vi "Calculate Distances.vi"(8 "error in (no error)":errorcluster, 11 "Grassfire in":refnum<class "Grassfire.lvclass">) -> (0 "error out":errorcluster, 3 "Grassfire out":refnum<class "Grassfire.lvclass">)   [LabVIEW 2019, in "Grassfire.lvclass"]
uses:
  Grassfire.lvclass
  Address/Address.lvclass
  Grassfire.lvclass/Grassfire.ctl
  Node/Node Value.lvclass
panel:
  out "i":i32
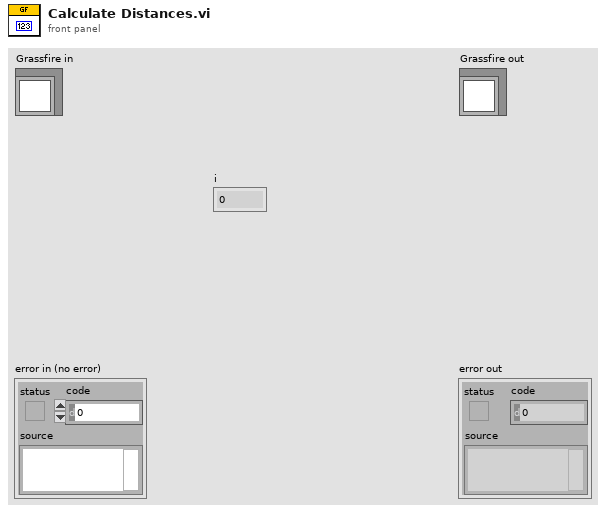
[diagram p1: front panel]
types:
  T1 = map{refnum<class "Address.lvclass">, refnum<class "Node Value.lvclass">}
  T2 = cluster{"Address":refnum<class "Address.lvclass">, "Step":i32}
  T3 = typedef "Node Value.lvclass/Node Type--enum.ctl" = enum16{"Empty", "Blocked", "Start", "End", "Path"}
  T4 = cluster{"2D Array Index":refnum<class "Address.lvclass">, i32}
  T5 = cluster{"Address":refnum<class "Address.lvclass">, "Step":i32}[]
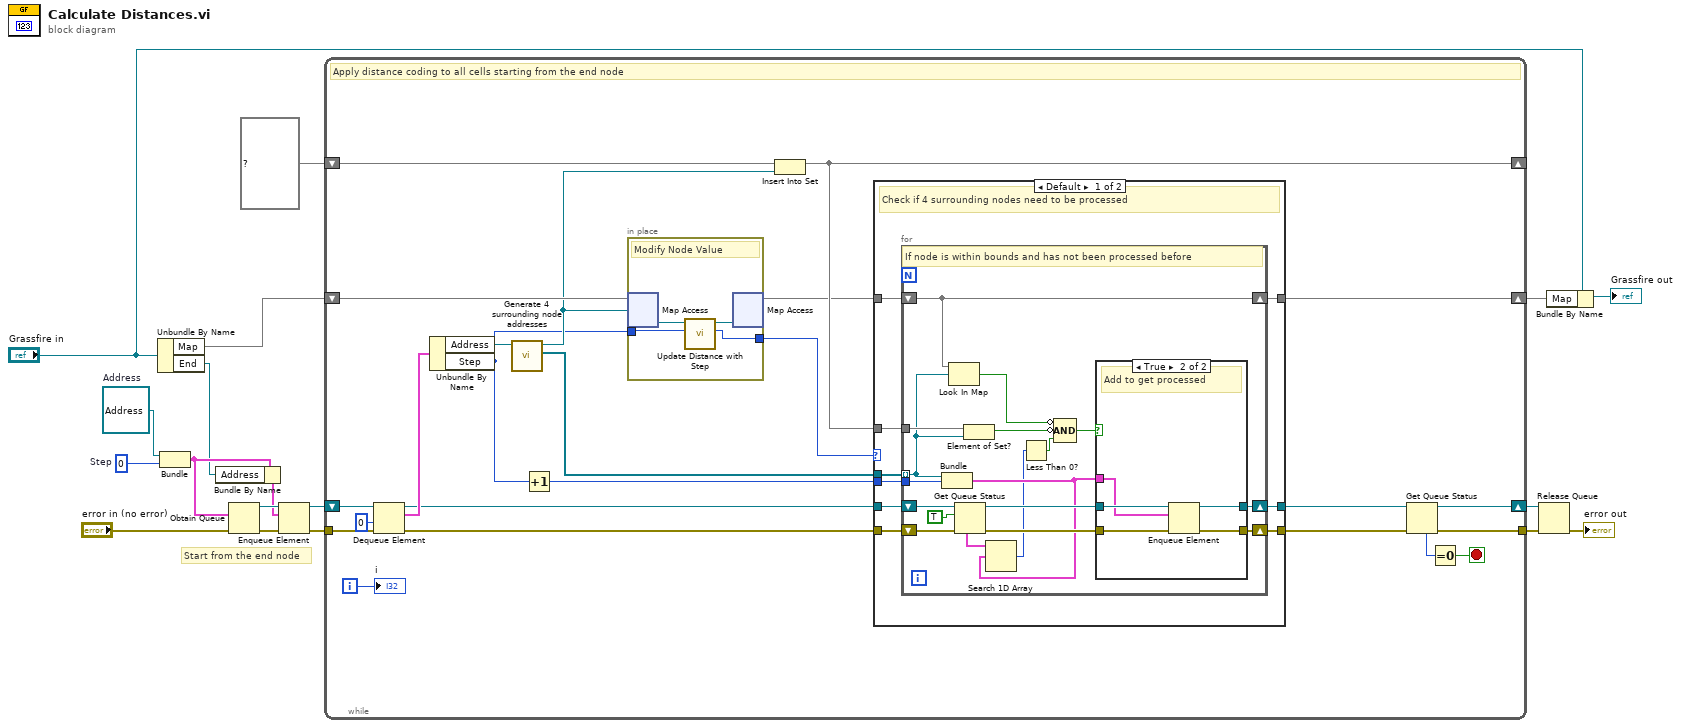
[diagram p0: block diagram]
diagram:
  w2 = refnum<class "Address.lvclass"> refnum  # Address
  w17 = 0  # Step
  # "Start from the end node"
  n1 = Unbundle By Name("Grassfire in") -> ("Map"=w12:T1, "End"=w14:refnum<class "Address.lvclass">)
  n2 = Bundle("Address"=w2, "Step"=w17) -> (w16:T2)  [unwired: 1 in]
  n3 = Bundle By Name(cluster=w16, "Address"=w14) -> (w15:T2)
  n4 = Obtain Queue(element data type=w16, error in (no error)="error in (no error)") -> (queue out=w18:refnum<queue>, error out=w9:errorcluster)  [unwired: 3 in, 1 out]
  n5 = Enqueue Element(queue=w18, element=w15, error in (no error)=w9) -> (queue out=w10:refnum<queue>, error out=w11:errorcluster)  [unwired: 1 in, 1 out]
  n6 = while {
    shift-right: [w42] -> w6
    shift-left: w12 -> [w25]
    shift-right: [w33] -> w4
    shift-left: w10 -> [w39]
    tunnel: w11 -> [w36]
    tunnel: [w34] -> w5
    shift-right: [w31] -> _
    shift-left: set{refnum<class "Address.lvclass">} {} ("set") -> [w32]
    i -> [w41]
    stop <- w30 stop-if-true
    # "Apply distance coding to all cells starting from the end node"
    n7 = Dequeue Element(queue=w39, timeout in ms (-1)=0, error in (no error)=w36) -> (queue out=w37:refnum<queue>, element=w38:T2, error out=w35:errorcluster)  [unwired: 1 out]
    n8 = Unbundle By Name(w38) -> ("Address"=w26:refnum<class "Address.lvclass">, "Step"=w20:i32)
    n9 = call "Generate 4 surrounding node addresses.vi"("2D Array in"=w26) -> ("4 Surrounding Nodes"=w23:refnum<class "Address.lvclass">[], "2D Array out"=w24:refnum<class "Address.lvclass">)  [unwired: 7 in, 2 out]
    n10 = Increment(x=w20) -> (x+1=w19:i32)
    n11 = in-place {
      in-place-border: w20 -> [w44]
      in-place-border: [w43] -> w22
      # "Modify Node Value"
      n12 = in-place-map #1(w25, w24) -> (w46:refnum<class "Node Value.lvclass">)  [unwired: 1 in, 1 out]
      n13 = call "Update Distance with Step.vi"("Step"=w44, "Picture Ring in"=w46) -> ("Node Type"=w43:T3, "Picture Ring out"=w45:refnum<class "Node Value.lvclass">)  [unwired: 7 in, 1 out]
      n14 = in-place-map #1(w45) -> (w21:T1)  [unwired: 1 in, 2 out]
    }
    n15 = Insert Into Set(10:w24, 11:w32) -> (3:w31:set{refnum<class "Address.lvclass">})  [unwired: 1 out]
    n16 = case shown="Default" w22 {
      tunnel: [w54 w82] -> w28
      tunnel: w23 -> [w53 _]
      tunnel: w37 -> [w55 w82]
      tunnel: w35 -> [w52 w81]
      tunnel: [w51 w81] -> w27
      tunnel: [w50 w83] -> w42
      tunnel: w21 -> [w49 w83]
      tunnel: w31 -> [w48 _]
      tunnel: w19 -> [w47 _]
      frame Default {
        # "Check if 4 surrounding nodes need to be processed"
        n17 = for {
          tunnel: w53 -> [w68] mode=indexing
          shift-right: [w73] -> w54
          shift-left: w55 -> [w65]
          shift-right: [w72] -> w51
          shift-left: w52 -> [w63]
          shift-right: [w66] -> w50
          shift-left: w49 -> [w66]
          tunnel: w48 -> [w69]
          tunnel: w47 -> [w59]
          # "If node is within bounds and has not been processed before"
          n18 = Bundle("2D Array Index"=w68, w59) -> (w58:T4)  [unwired: 1 in]
          n19 = Look In Map(map=w66, key=w68) -> (key not found?=w71:bool)  [unwired: 1 in, 1 out]
          n20 = Get Queue Status(queue=w65, return elements? (F)=TRUE, error in (no error)=w63) -> (queue out=w62:refnum<queue>, error out=w61:errorcluster, elements=w60:T5)  [unwired: 5 out]
          n21 = Element of Set?(10:w68, 11:w69) -> (3:w67:bool)
          n22 = Search 1D Array(1D array=w60, element=w58) -> (index of element=w56:i32)  [unwired: 1 in]
          n23 = Less Than 0?(x=w56) -> (x < 0?=w57:bool)
          n24 = Compound Arithmetic op=AND(invert w71, invert w67, w57) -> (w70:bool)
          n25 = case shown="True" w70 {
            tunnel: w62 -> [w75 w80]
            tunnel: [w75 w79] -> w73
            tunnel: w61 -> [w74 w78]
            tunnel: [w74 w77] -> w72
            tunnel: w58 -> [_ w76]
            frame False {
              # "Ignore node"
            }
            frame True {
              # "Add to get processed"
              n26 = Enqueue Element(queue=w80, element=w76, error in (no error)=w78) -> (queue out=w79:refnum<queue>, error out=w77:errorcluster)  [unwired: 1 in, 1 out]
            }
          }
        }
      }
      frame "Blocked" {
        # "No further actions"
      }
    }
    n27 = Get Queue Status(queue=w28, error in (no error)=w27) -> (queue out=w33:refnum<queue>, error out=w34:errorcluster, # elements in queue=w29:i32)  [unwired: 1 in, 5 out]
    n28 = Equal To 0?(x=w29) -> (x = 0?=w30:bool)
    "i" <- w41
  }
  n29 = Release Queue(queue=w4, error in (no error)=w5) -> (error out=→"error out":errorcluster)  [unwired: 1 in, 2 out]
  n30 = Bundle By Name(cluster="Grassfire in", "Map"=w6) -> (→"Grassfire out":refnum<class "Grassfire.lvclass">)
